vi "Update Kitchen Table Step Done by Index.vi"(8 "error in (no error)":errorcluster, 11 "Cooker Actor in":refnum<class "Cooker Actor.lvclass">) -> (0 "error out":errorcluster, 3 "Cooker Actor out":refnum<class "Cooker Actor.lvclass">)   [LabVIEW 2024, in "Cooker Actor.lvlib" / "Cooker Actor.lvclass"]
uses:
  Cooker Actor.lvclass
  C:/Program Files/National Instruments/LabVIEW 2024/vi.lib/ActorFramework/Actor/Actor.lvclass
  <vilib>/ActorFramework/Actor/Actor.lvclass/Actor.ctl
  Cooker Actor.lvclass/Cooker Actor.ctl
  Kitchen Messaging Interface/Kitchen Messaging Interface Messages/Update Table Step Done by Index Msg/Update Table Step Done by Index Msg.lvclass/Update Table Step Done by Index Msg.ctl
  <vilib>/ActorFramework/Message Enqueuer/Message Enqueuer.lvclass/Message Enqueuer.ctl
  Kitchen Messaging Interface/Kitchen Messaging Interface Messages/Dye Recipe Table Step by Index Msg/Dye Recipe Table Step by Index Msg.lvclass/Dye Recipe Table Step by Index Msg.ctl
  <vilib>/ActorFramework/Message Enqueuer/Init from Existing Queue.vi
  <vilib>/ActorFramework/Message Enqueuer/Enqueue.vi
  Kitchen Messaging Interface/Kitchen Messaging Interface Messages/Update Table Step Done by Index Msg/Update Table Step Done by Index Msg.lvclass
  C:/Program Files/National Instruments/LabVIEW 2024/vi.lib/ActorFramework/Message/Message.lvclass
  Kitchen Messaging Interface/Kitchen Messaging Interface Messages/Dye Recipe Table Step by Index Msg/Dye Recipe Table Step by Index Msg.lvclass
  <vilib>/ActorFramework/Message Priority Queue/Priority Enqueue.vi
  <vilib>/ActorFramework/Message Enqueuer/Message Enqueuer.lvclass
  Support/Recipe/Recipe.lvclass
  <vilib>/ActorFramework/Actor/Actor.lvclass
  Cooker Actor Messages/Stop Cooking Msg/Stop Cooking Msg.lvclass
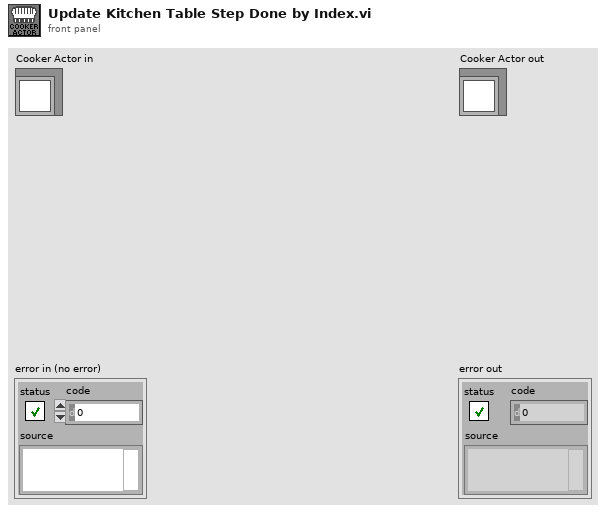
[diagram p1: front panel]
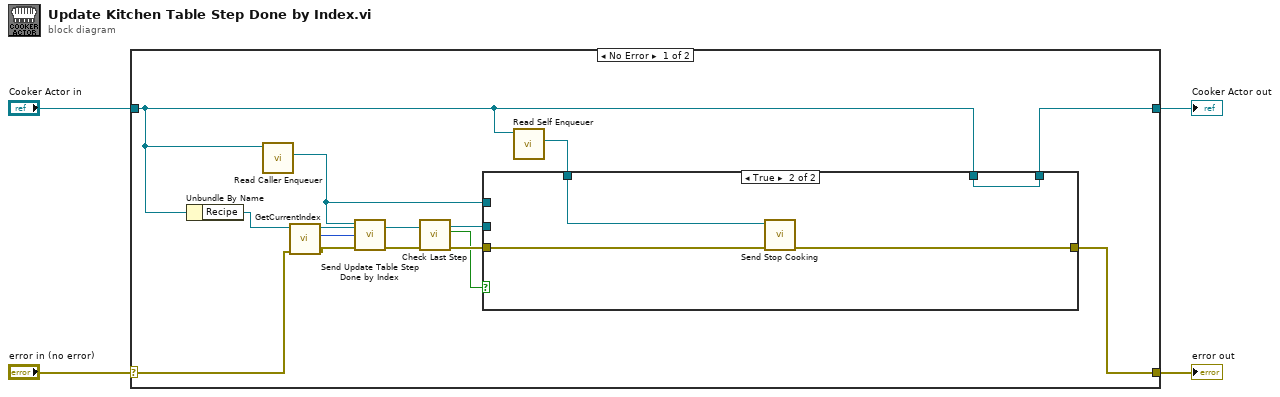
[diagram p0: block diagram]
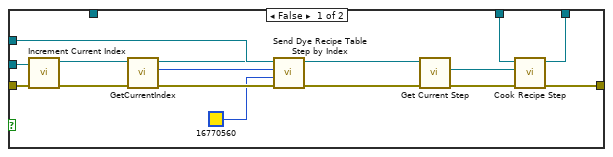
[diagram p2: hidden frame]
diagram:
  n1 = case shown="No Error" "error in (no error)" {
    selector: "error in (no error)" -> [w14 w38]
    tunnel: [w12 w38] -> w3
    tunnel: [w8 w37] -> w1
    tunnel: "Cooker Actor in" -> [w6 w37]
    frame No Error {
      n2 = Unbundle By Name(w6) -> ("Recipe"=w16:refnum<class "Recipe.lvclass">)
      n3 = call <vilib>:"Read Caller Enqueuer.vi"("Actor"=w6) -> ("Caller Enqueuer"=w7:refnum<class "Message Enqueuer.lvclass">)  [unwired: 10 in]
      n4 = call-dynamic "GetCurrentIndex.vi"("Error In"=w14, "reference in"=w16) -> ("Error Out"=w13:errorcluster, "Current Index"=w15:u64, "reference out"=w11:refnum<class "Recipe.lvclass">)  [unwired: 7 in]
      n5 = call "Send Update Table Step Done by Index.vi"("error in (no error)"=w13, "Index"=w15, "Message Enqueuer"=w7) -> ("error out"=w17:errorcluster)  [unwired: 7 in, 1 out]
      n6 = call-dynamic "Check Last Step.vi"("reference in"=w11) -> ("Is Last Step"=w9:bool, "reference out"=w10:refnum<class "Recipe.lvclass">)  [unwired: 8 in, 1 out]
      n7 = call <vilib>:"Read Self Enqueuer.vi"("Actor"=w6) -> ("Self Enqueuer"=w5:refnum<class "Message Enqueuer.lvclass">)  [unwired: 10 in]
      n8 = case shown="True" w9 {
        tunnel: w17 -> [w32 w36]
        tunnel: [w28 w34] -> w12
        tunnel: w10 -> [w30 _]
        tunnel: w6 -> [w27 w35]
        tunnel: [w26 w35] -> w8
        tunnel: w7 -> [w21 _]
        tunnel: w5 -> [_ w33]
        frame False {
          n9 = call-dynamic "Increment Current Index.vi"("Error In"=w32, "reference in"=w30) -> ("Error Out"=w31:errorcluster, "reference out"=w23:refnum<class "Recipe.lvclass">)  [unwired: 8 in]
          n10 = call-dynamic "GetCurrentIndex.vi"("Error In"=w31, "reference in"=w23) -> ("Error Out"=w24:errorcluster, "Current Index"=w19:u64, "reference out"=w20:refnum<class "Recipe.lvclass">)  [unwired: 7 in]
          n11 = call "Send Dye Recipe Table Step by Index.vi"("error in (no error)"=w24, "Dye Color"=u32 16770560, "Index"=w19, "Message Enqueuer"=w21) -> ("error out"=w22:errorcluster)  [unwired: 6 in, 1 out]
          n12 = call-dynamic "Get Current Step.vi"("error in (no error)"=w22, "Recipe in"=w20) -> ("error out"=w29:errorcluster, "Recipe Step"=w25:refnum<class "Recipe Step.lvclass">)  [unwired: 7 in, 1 out]
          n13 = call-dynamic "Cook Recipe Step.vi"("error in (no error)"=w29, "Recipe Step"=w25, "Cooker Actor in"=w27) -> ("error out"=w28:errorcluster, "Cooker Actor out"=w26:refnum<class "Cooker Actor.lvclass">)  [unwired: 7 in]
        }
        frame True {
          n14 = call "Send Stop Cooking.vi"("error in (no error)"=w36, "Message Enqueuer"=w33) -> ("error out"=w34:errorcluster)  [unwired: 8 in, 1 out]
        }
      }
    }
    frame Error {
    }
  }
  "error out" <- w3
  "Cooker Actor out" <- w1
